vi "simple checkpoint.vi"(9 "Current location":cluster{"x":i16, "y":i16}, 11 "checkpoint queue":refnum<queue>) -> (2 "next checkpoint":T1)   [LabVIEW 2009]
uses:
  object.ctl
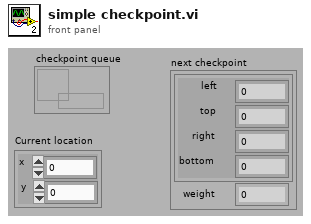
[diagram p1: front panel]
types:
  T1 = typedef "object.ctl" = cluster{"rect":cluster{"left":i16, "top":i16, "right":i16, "bottom":i16}, "weight":sgl}
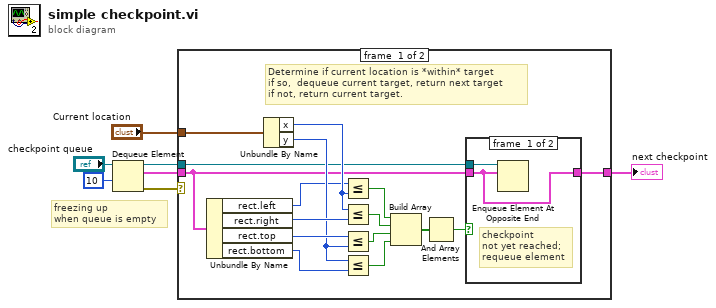
[diagram p0: block diagram]
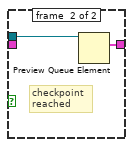
[diagram p2: hidden frame]
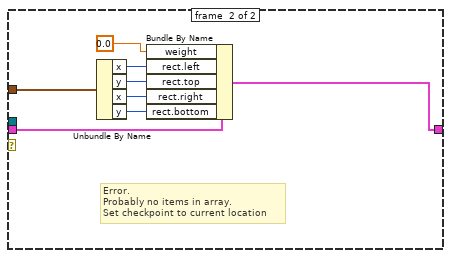
[diagram p3: hidden frame]
diagram:
  # "freezing up\nwhen queue is empty"
  n1 = Dequeue Element(queue="checkpoint queue", timeout in ms (-1)=10) -> (queue out=w5:refnum<queue>, element=w3:T1, error out=w1:errorcluster)  [unwired: 1 in, 1 out]
  n2 = case shown="No Error" w1 {
    tunnel: "Current location" -> [w23 w34]
    tunnel: w5 -> [w11 _]
    tunnel: [w10 w28] -> w4
    tunnel: w3 -> [w8 w35]
    frame #0 {
      # "Determine if current location is *within* target\nif so,  dequeue current target, return next target\nif not, return current target."
      n3 = Unbundle By Name(w8) -> ("rect.left"=w18:i16, "rect.right"=w21:i16, "rect.top"=w20:i16, "rect.bottom"=w17:i16)
      n4 = Unbundle By Name(w23) -> ("x"=w22:i16, "y"=w19:i16)
      n5 = Less Or Equal?(x=w18, y=w22) -> (x <= y?=w16:bool)
      n6 = Less Or Equal?(x=w22, y=w21) -> (x <= y?=w15:bool)
      n7 = Less Or Equal?(x=w20, y=w19) -> (x <= y?=w13:bool)
      n8 = Less Or Equal?(x=w19, y=w17) -> (x <= y?=w14:bool)
      n9 = Build Array(w16, w15, w13, w14) -> (w12:bool[])
      n10 = And Array Elements(Boolean array=w12) -> (logical AND=w9:bool)
      n11 = case shown="False" w9 {
        tunnel: w11 -> [w25 w26]
        tunnel: [w24 w27] -> w10
        tunnel: w8 -> [w24 _]
        frame #0 {
          # "checkpoint\nnot yet reached;\nrequeue element"
          n12 = Enqueue Element At Opposite End(queue=w25, element=w24) -> ()  [unwired: 2 in, 3 out]
        }
        frame #1 {
          # "checkpoint\nreached"
          n13 = Preview Queue Element(queue=w26) -> (element=w27:T1)  [unwired: 2 in, 3 out]
        }
      }
    }
    frame #1 {
      # "Error.\nProbably no items in array.\nSet checkpoint to current location"
      n14 = Unbundle By Name(w34) -> ("x"=w33:i16, "y"=w32:i16, "x"=w31:i16, "y"=w30:i16)
      n15 = Bundle By Name(cluster=w35, "weight"=sgl 0.0, "rect.left"=w33, "rect.top"=w32, "rect.right"=w31, "rect.bottom"=w30) -> (w28:T1)
    }
  }
  "next checkpoint" <- w4
